vi "Triggers-Start.vi"(7 "Setup/Logging queue element":T1={"Imaging Protocol"=enum."Live Imaging", "Number of Trials"=0, "Frame Size"=512, "# Averaged frames"=0, "Dwell time (us)"=0.0, "Index of Z-plane"=0, "Timelapse?"=FALSE, "Logging process is active"=FALSE, "Speed logging enabled"=FALSE, "tdms file ref"=refnum, "path"=path "", "Trial Number"=0, "Expected # points acquired"=FALSE, "Manually stopped"=FALSE, "Last trial"=FALSE, "Ch0 data"=[], "Ch1 data"=[], "Ref Data"=[], "Ref Frame Time"=[], "Image Time"=[], "Continuous Time"=[], "Ref X Length"=0, "Ref Y Length"=0, "# Ref Averaged frames"=0, "Ref Dwell time (us)"=0.0, "Points acquired"={"Ch0 last trial"=0, "Ch1 last trial"=0, "All trials"=0}, "HW Timings File"=refnum} {"Ref Dwell time (us)" format="%#.6g"; "Frame Size" items=["100X100"=100, "128X128"=128, "200X200"=200, "256X256"=256, "512X512"=512, "1024x1024"=1024, "2048x2048"=2048]; "Dwell time (us)" format="%#.6g"}, 8 "error in (no error)":errorcluster, 11 "FPGA Ref":T5) -> (0 "error out":errorcluster)   [LabVIEW 2017]
uses:
  RIG-SPECIFIC FILES/FPGA Refs/FPGA Ref.ctl
  Typedefs/Logging queue element.ctl
  Typedefs/Imaging Protocols enum.ctl
  Typedefs/Frame Size.ctl
  Typedefs/Acquired points count.ctl
  Typedefs/HW config states enum.ctl
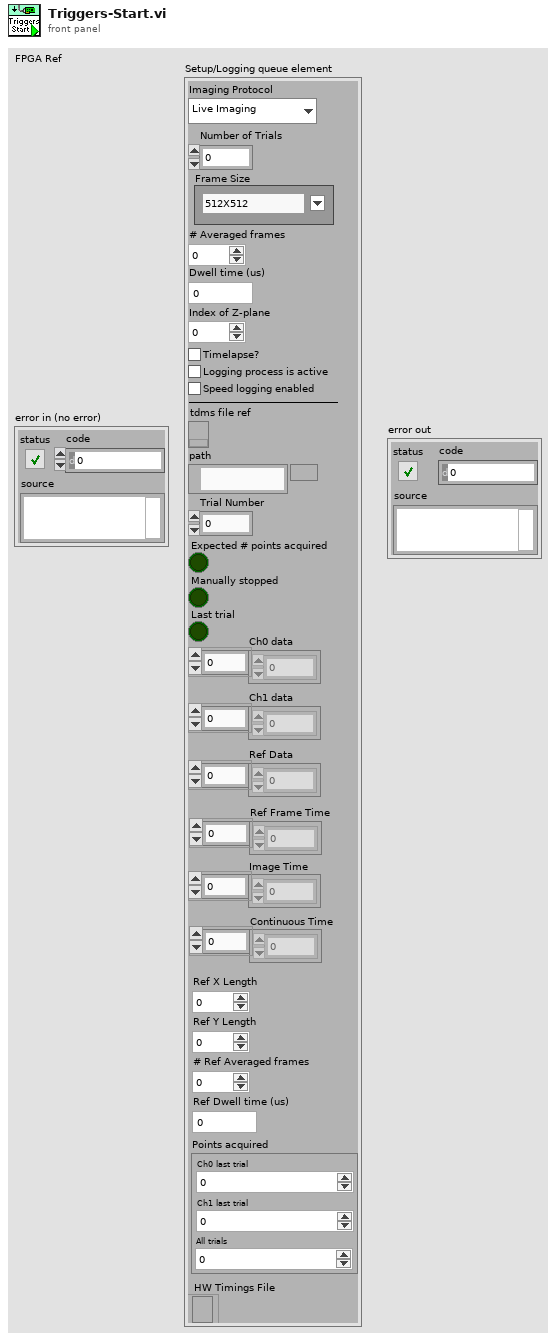
[diagram p1: front panel]
types:
  T1 = typedef "Logging queue element.ctl" = cluster{"Imaging Protocol":T2, "Number of Trials":u16, "Frame Size":T3, "# Averaged frames":u16, "Dwell time (us)":dbl, "Index of Z-plane":i32, "Timelapse?":bool, "Logging process is active":bool, "Speed logging enabled":bool, "tdms file ref":refnum<k34>, "path":path, "Trial Number":i32, "Expected # points acquired":bool, "Manually stopped":bool, "Last trial":bool, "Ch0 data":u32[], "Ch1 data":u32[], "Ref Data":u32[], "Ref Frame Time":u64[], "Image Time":u64[], "Continuous Time":u64[], "Ref X Length":u16, "Ref Y Length":u16, "# Ref Averaged frames":u16, "Ref Dwell time (us)":dbl, "Points acquired":T4, "HW Timings File":refnum<file>}
  T2 = typedef "Imaging Protocols enum.ctl" = enum16{"AOL Z-Stack", "Motor Z Stack", "Functional Acquisition", "Single Plane Acquisition", "Volume Acquisition", "Live Imaging", "Live Plane Imaging", "Live Volume Imaging"}
  T3 = typedef "Frame Size.ctl" = u16
  T4 = typedef "Acquired points count.ctl" = cluster{"Ch0 last trial":u64, "Ch1 last trial":u64, "All trials":u64}
  T5 = typedef "FPGA Ref.ctl" = refnum<k20>
  T6 = typedef "HW config states enum.ctl" = enum16{"Load from file", "Save to file", "Write all", "Read all", "Write XY stage settings", "Write DAQ FPGA settings", "Write Control FPGA settings", "Write Phys Channels", "Write System Config", "Write HW Config", "Save System Config", "Save HW Config", "Clear", "Compare from file"}
  T7 = typedef "Hardware Configuration settings.ctl" = cluster{"Dev. PC":bool, "Swap XY on stage":bool, "No of AOD":u8, "MC Supported":bool, "Axial MC":bool, "Computer MAC address":string, "Externalise Triggers":bool, "Trigger HW config":T8, "DAQmx Chan":T9, "XY stage available":bool, "XY Stage":T10, "Z stage available":bool, "Z Stage config cluster":T11, "Encoder available":bool, "Encoder":T12, "VidRec available":bool, "Cam VidRec":T13, "Laser Power Control HW config":T14, "Laser 1 available":bool, "Laser 1 config cluster":T15, "Prechirper 1 available":bool, "Prechirper 1 config cluster":T16, "Control system.FPGA available?":bool, "Control Sys. HW config":T17, "DAQ FPGA HW Config":T18}
  T8 = typedef "Triggers HW config.ctl" = cluster{"Available Device List":i32, "Device Address":string}
  T9 = typedef "DAQmx physical channels cluster.ctl" = cluster{"Pockels AO":tag, "Hard shutter AO":tag, "PMT AOs":tag, "Galvo AOs":tag, "Power meter AI":tag}
  T10 = typedef "XY Stage config cluster.ctl" = cluster{"COM port":refnum<visa-resource-name>, "Baudrate":i32, "Type":string}
  T11 = typedef "Z Stage config cluster.ctl" = cluster{"COM port":refnum<visa-resource-name>, "Baudrate":i32, "Type":string}
  T12 = typedef "Encoder config cluster.ctl" = cluster{"IP address":string, "Port":u16, "Wheel radius (cm)":dbl, "Encoder Trigger":tag}
  T13 = typedef "Cam VidRec HW config setup cluster.ctl" = cluster{"DO flag-Video record":tag, "DO flag-Trial start":tag}
  T14 = typedef "Laser Power Control HW config.ctl" = cluster{"Laser Power Control":string, "Laser Power Modulation Control":enum16{"NI", "FPGA"}}
  T15 = typedef "Laser 1 config cluster.ctl" = cluster{"COM port":refnum<visa-resource-name>, "Baud Rate":i32, "Type":string}
  T16 = typedef "PreChirper 1 config cluster.ctl" = cluster{"Type":string, "Baud Rate":i32, "COM port":refnum<visa-resource-name>}
  T17 = typedef "Control Sys HW config cluster.ctl" = cluster{"Control system.FPGA Type":enum16{"Virtex 5", "Virtex 7"}, "Control system.Network adapter name":string, "Control system.MAC address":string, "Control system.Ethernet Port":u32, "Control system.Ethernet Port Opened":bool}
  T18 = typedef "DAQ FPGA HW config cluster.ctl" = cluster{"FGPA Ref":T5, "Target":T19, "input card type":T20}
  T19 = typedef "nirio_resource_hc.ctl" = tag
  T20 = typedef "FPGA input type AC-DC.ctl" = enum16{"AC Card", "DC Card"}
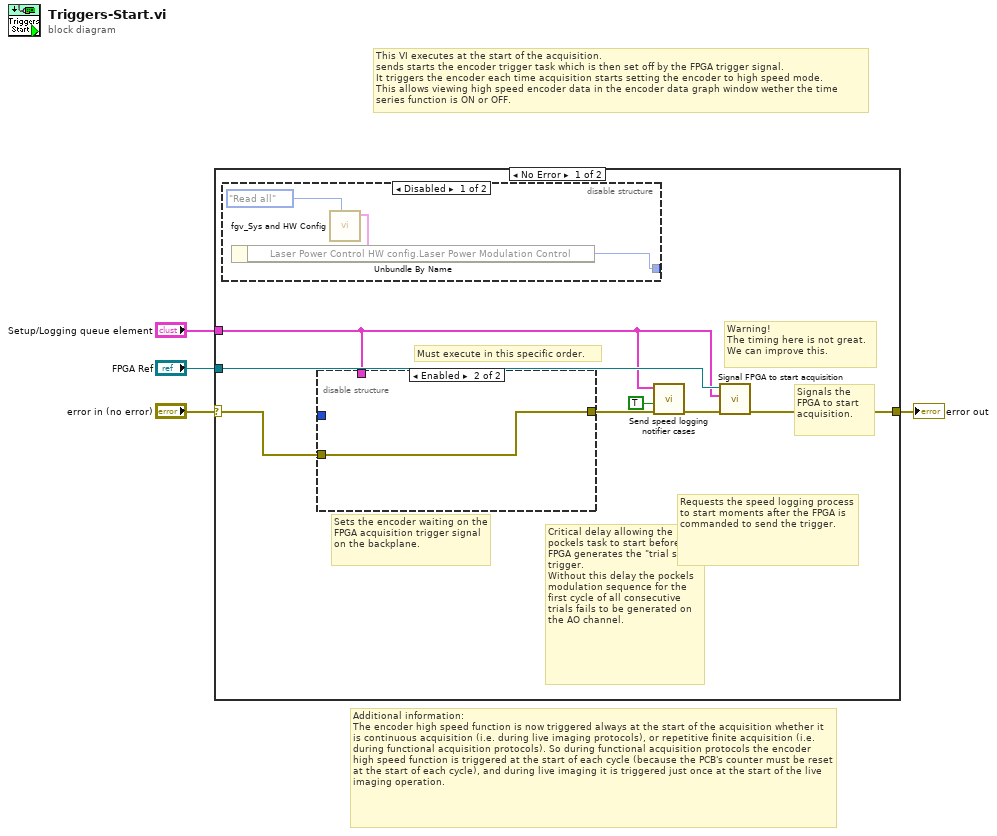
[diagram p0: block diagram]
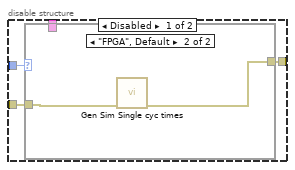
[diagram p3: hidden frame]
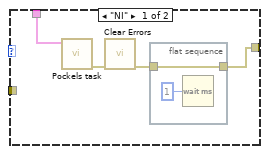
[diagram p4: hidden frame]
diagram:
  # "Additional information:\nThe encoder high speed function is now triggered always at the start of the acquisition whether it is continuous acquisition (i.e. during live imaging protocols), or repetitive finite acquisition (i.e. during functional acquisition protocols). So during functional acquisition protocols the encoder high speed function is triggered at the start of each cycle (because the PCB's counter must be reset at the start of each cycle), and during live imaging it is triggered just once at the start of the live imaging operation."
  # "This VI executes at the start of the acquisition.\nsends starts the encoder trigger task which is then set off by the FPGA trigger signal.\nIt triggers the encoder each time acquisition starts setting the encoder to high speed mode.\nThis allows viewing high speed encoder data in the encoder data graph window wether the time series function is ON or OFF."
  n1 = case shown="No Error" "error in (no error)" {
    selector: "error in (no error)" -> [w5 w28]
    tunnel: "FPGA Ref" -> [w11 _]
    tunnel: [w6 w28] -> w3
    tunnel: "Setup/Logging queue element" -> [w9 _]
    frame No Error {
      # "Critical delay allowing the pockels task to start before the FPGA generates the \"trial start\" trigger.\nWithout this delay the pockels modulation sequence for the first cycle of all consecutive trials fails to be generated on the AO channel."
      # "Warning!\nThe timing here is not great.\nWe can improve this."
      # "Requests the speed logging process to start moments after the FPGA is commanded to send the trigger."
      # "Signals the FPGA to start acquisition."
      # "Sets the encoder waiting on the FPGA acquisition trigger signal on the backplane."
      # "Must execute in this specific order."
      n2 = disable-structure shown="Disabled" {
        disable-tunnel: [w12 _] -> _
        frame Disabled {
          n3 = call "fgv_Sys and HW Config.vi"("Function"=HW_config_states_enum."Read all") -> ("Hardware Configuration OUT"=w13:T7)  [unwired: 8 in, 2 out]
          n4 = Unbundle By Name(w13) -> ("Laser Power Control HW config.Laser Power Modulation Control"=w12:enum16{"NI", "FPGA"})
        }
        frame Enabled {
        }
      }
      n5 = disable-structure shown="Enabled" {
        disable-tunnel: w9 -> [w18 _]
        disable-tunnel: [w17 w27] -> w8
        disable-tunnel: w5 -> [w16 w27]
        disable-tunnel: _ -> [w15 _]
        frame Disabled {
          n6 = case shown="\"FPGA\", Default" w15 {
            tunnel: w18 -> [w22 _]
            tunnel: [w21 w25] -> w17
            tunnel: w16 -> [_ w26]
            frame "NI" {
              n7 = call "Pockels task.vi"("Setup/Logging queue element"=w22) -> ("error out"=w20:errorcluster)  [unwired: 10 in]
              n8 = call <vilib>:"Clear Errors.vi"("error in (no error)"=w20) -> ("error out"=w19:errorcluster)  [unwired: 5 in, 1 out]
              n9 = flat-sequence {
                tunnel: [w23] -> w21
                tunnel: w19 -> [w23]
                frame #0 {
                  n10 = Wait (ms)(milliseconds to wait=u32 1) -> ()  [unwired: 1 out]
                }
              }
            }
            frame "FPGA", Default {
              n11 = call "Gen Sim Single cyc times.vi"("error in (no error)"=w26) -> ("error out"=w25:errorcluster)  [unwired: 10 in]
            }
          }
        }
        frame Enabled {
        }
      }
      n12 = call "Send speed logging notifier cases.vi"("error in"=w8, "Log speed data = T (Unused)"=TRUE ("Log speed data"), "Setup/Logging queue element"=w9) -> ("error out"=w7:errorcluster)  [unwired: 8 in]
      n13 = call "Signal FPGA to start acquisition.vi"("error in (no error)"=w7, "Logging queue element"=w9, "FPGA VI Ref"=w11) -> ("error out"=w6:errorcluster)  [unwired: 7 in, 1 out]
    }
    frame Error {
    }
  }
  "error out" <- w3
